vi "Initialize.vi"(7 "Custom Device Name":string, 8 "error in":errorcluster, 9 "Compiled Settings":variant, 10 "Custom Device API in":refnum<class "Custom Device API.lvclass">, 11 "Custom Device In":refnum<class "Custom Device.lvclass">) -> (0 "error out":errorcluster, 3 "Custom Device out":refnum<class "Custom Device.lvclass">)   [LabVIEW 2027, in "Custom Device Interfaces.lvlib" / "Custom Device.lvclass"]
uses:
  Custom Device.lvclass
  CustomDeviceAPI/Custom Device API.lvclass
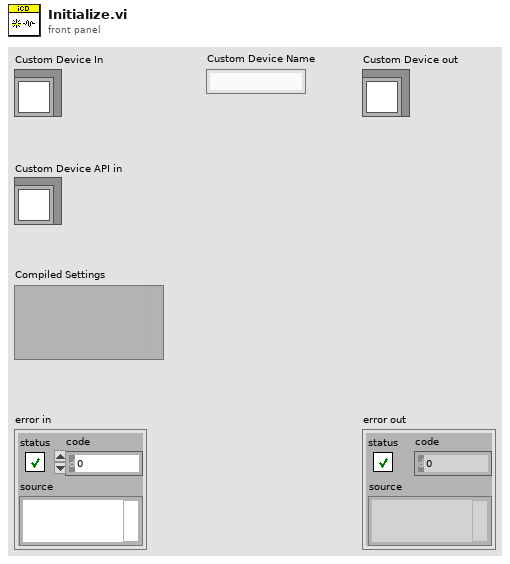
[diagram p1: front panel]
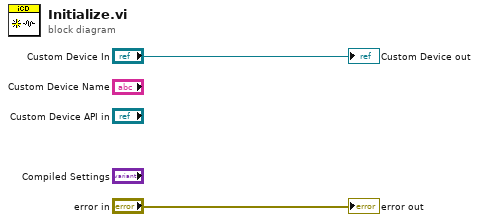
[diagram p0: block diagram]
diagram:
  "error out" <- "error in"
  "Custom Device out" <- "Custom Device In"
